vi "Query Multi Eval Meas List Segment Bandwidth Part.vi"(6 "Segment (1)":T3=1, 7 "Bandwidth Part (BWP0)":T1 items=["BWP0"], 8 "error in (no error)":errorcluster, 9 "Carrier Component (1)":T2=1, 10 "Instance (1)":T4=1, 11 "VISA resource name":refnum<visa-resource-name>) -> (0 "error out":errorcluster, 1 "Cyclic Prefix":i32(ring) items=["Normal"], 2 "No Of RBs":i32=66, 3 "VISA resource name out":refnum<visa-resource-name>, 4 "Start RB":i32, 5 "Subcarrier Spacing":i32(ring)=1 items=["60 kHz", "120 kHz"])   [LabVIEW 2020, in "Rohde&Schwarz CMXP NR FR2 Measurement.lvlib"]
doc: "Queries basic properties of the <BWP> on carrier <cc> in segment <no>.\n\nAttribute:\n-\n\nRemote-control command:\nCONFigure:NRMMw:MEAS<i>:LIST:SEGMent<no>[:CC<cc>]:BWPart? <BWP>"
uses:
  <instrlib>/Rohde&Schwarz CMXP NR FR2 Measurement/Rohde&Schwarz CMXP NR FR2 Measurement.lvlib
  <instrlib>/Rohde&Schwarz CMXP NR FR2 Measurement/Private/_Instance.ctl
  <instrlib>/Rohde&Schwarz CMXP NR FR2 Measurement/Private/_Segment.ctl
  <instrlib>/Rohde&Schwarz CMXP NR FR2 Measurement/Private/_Carrier Component.ctl
  <instrlib>/Rohde&Schwarz CMXP NR FR2 Measurement/Private/_Bandwidth Part.ctl
  <instrlib>/Rohde&Schwarz CMXP NR FR2 Measurement/Private/rsidr_core.llb/rsidr_core.lvlib
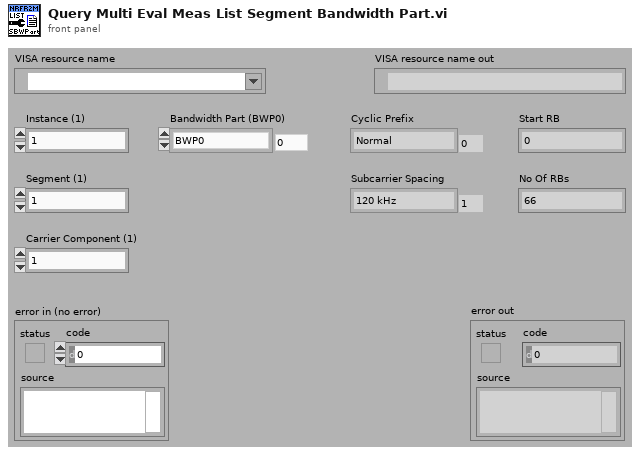
[diagram p1: front panel]
types:
  T1 = typedef "Rohde&Schwarz CMXP NR FR2 Measurement.lvlib/_Bandwidth Part.ctl" = i32
  T2 = typedef "Rohde&Schwarz CMXP NR FR2 Measurement.lvlib/_Carrier Component.ctl" = i32
  T3 = typedef "Rohde&Schwarz CMXP NR FR2 Measurement.lvlib/_Segment.ctl" = i32
  T4 = typedef "Rohde&Schwarz CMXP NR FR2 Measurement.lvlib/_Instance.ctl" = i32
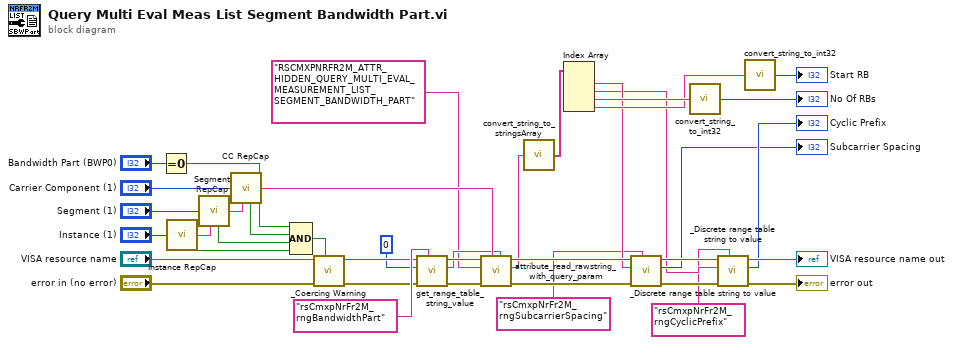
[diagram p0: block diagram]
diagram:
  n1 = Equal To 0?(x="Bandwidth Part (BWP0)") -> (x = 0?=w9:bool)
  n2 = call <instrlib>:"Instance RepCap.vi"("Instance In"="Instance (1)") -> ("In Range?"=w35:bool, "RepCap Identifier Out"=w7:string)  [unwired: 1 in]
  n3 = call <instrlib>:"Segment RepCap.vi"("Segment In"="Segment (1)", "RepCap String In (\"\")"=w7) -> ("In Range?"=w34:bool, "RepCap Identifier Out"=w32:string)
  n4 = call <instrlib>:"CC RepCap.vi"("CC In"="Carrier Component (1)", "RepCap String In (\"\")"=w32) -> ("In Range?"=w33:bool, "RepCap Identifier Out"=w21:string)
  n5 = Compound Arithmetic op=AND(w9, w33, w34, w35) -> (w38:bool)
  n6 = call <instrlib>:"_Coercing Warning.vi"("In Range?"=w38, "error in (no error)"="error in (no error)", "VISA resource name"="VISA resource name") -> ("error out"=w28:errorcluster, "VISA resource name out"=w29:refnum<visa-resource-name>)  [unwired: 7 in]
  n7 = call <instrlib>:"get_range_table_string_value.vi"("Range Table ID in"="rsCmxpNrFr2M_rngBandwidthPart", "error in"=w28, "I32 input"=0, "VISA resource name"=w29) -> ("error out"=w23:errorcluster, "String Value out"=w20:string, "VISA resource name out"=w22:refnum<visa-resource-name>)  [unwired: 5 in]
  n8 = call <instrlib>:"attribute_read_rawstring_with_query_param.vi"("Query Parameter (None)"=w20, "Repeated Capability"=w21, "error in"=w23, "Attribute ID"="RSCMXPNRFR2M_ATTR_HIDDEN_QUERY_MULTI_EVAL_MEASUREMENT_LIST_SEGMENT_BANDWIDTH_PART", "VISA resource name"=w22) -> ("error out"=w27:errorcluster, "Raw String out"=w13:string, "VISA resource name out"=w25:refnum<visa-resource-name>)  [unwired: 4 in]
  n9 = call <instrlib>:"convert_string_to_stringsArray.vi"("String in"=w13) -> ("string array out"=w14:string[])  [unwired: 3 in, 1 out]
  n10 = Index Array(array=w14) -> (element #1=w4:string, element #2=w3:string, element #3=w24:string, element #4=w5:string)  [unwired: 4 in]
  n11 = call <instrlib>:"_Discrete range table string to value.vi"("Discrete Range Table Identifier"="rsCmxpNrFr2M_rngSubcarrierSpacing", "error in (no error)"=w27, "String Value In"=w4, "VISA resource name"=w25) -> ("error out"=w26:errorcluster, "Enum Value"=→"Subcarrier Spacing":i32, "VISA resource name out"=w12:refnum<visa-resource-name>)  [unwired: 5 in]
  n12 = call <instrlib>:"convert_string_to_int32.vi"("String in"=w24) -> ("int32 value out"=→"No Of RBs":i32)  [unwired: 4 in]
  n13 = call <instrlib>:"_Discrete range table string to value.vi"("Discrete Range Table Identifier"="rsCmxpNrFr2M_rngCyclicPrefix", "error in (no error)"=w26, "String Value In"=w3, "VISA resource name"=w12) -> ("error out"=→"error out":errorcluster, "Enum Value"=→"Cyclic Prefix":i32, "VISA resource name out"=→"VISA resource name out":refnum<visa-resource-name>)  [unwired: 5 in]
  n14 = call <instrlib>:"convert_string_to_int32.vi"("String in"=w5) -> ("int32 value out"=→"Start RB":i32)  [unwired: 4 in]
